vi "Confirm Hardware Found.vi"(8 "error in":errorcluster, 11 "HW Config":T1) -> (0 "error out":errorcluster, 3 "Configure Hardware?":bool)   [LabVIEW 2020, in "SEECD System Explorer.lvlib"]
uses:
  SEECD System Explorer.lvlib
  Type Defs/Host - HW Config.ctl
  Type Defs/Host - Local Chassis.ctl
  Type Defs/Host - Module.ctl
  Type Defs/IOV Container Contents.ctl
  Type Defs/Host - Master.ctl
  Type Defs/Host - Slave.ctl
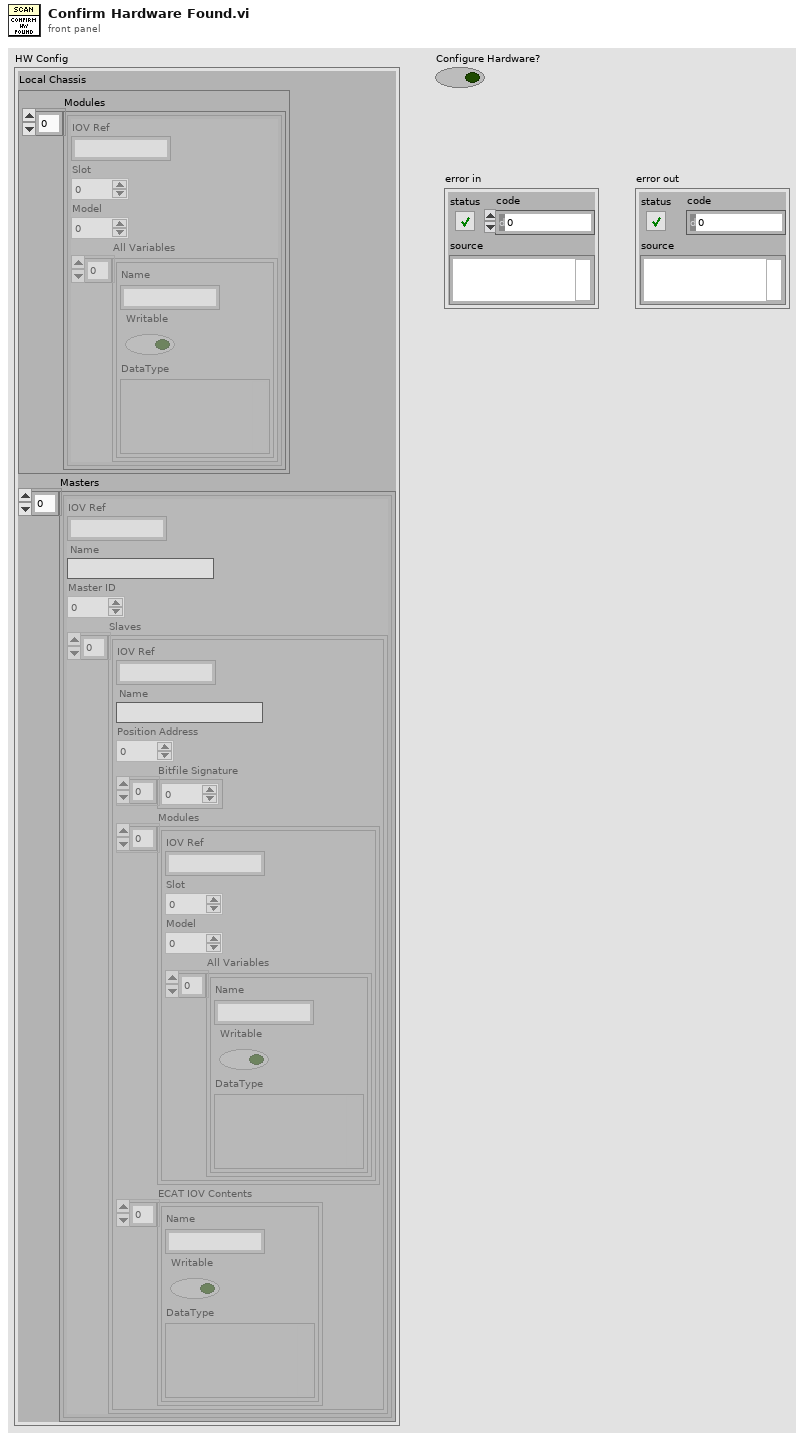
[diagram p1: front panel]
types:
  T1 = typedef "SEECD System Explorer.lvlib/Host - HW Config.ctl" = cluster{"Local Chassis":T2, "Masters":T5[]}
  T2 = typedef "SEECD System Explorer.lvlib/Host - Local Chassis.ctl" = cluster{"Modules":T3[]}
  T3 = typedef "SEECD System Explorer.lvlib/Host - Module.ctl" = cluster{"IOV Ref":string, "Slot":u32, "Model":u32, "All Variables":T4[]}
  T4 = typedef "SEECD System Explorer.lvlib/IOV Container Contents.ctl" = cluster{"Name":string, "Writable":bool, "DataType":variant}
  T5 = typedef "SEECD System Explorer.lvlib/Host - Master.ctl" = cluster{"IOV Ref":string, "Name":string, "Master ID":u32, "Slaves":T6[]}
  T6 = typedef "SEECD System Explorer.lvlib/Host - Slave.ctl" = cluster{"IOV Ref":string, "Name":string, "Position Address":u16, "Bitfile Signature":u8[], "Modules":T3[], "ECAT IOV Contents":T4[]}
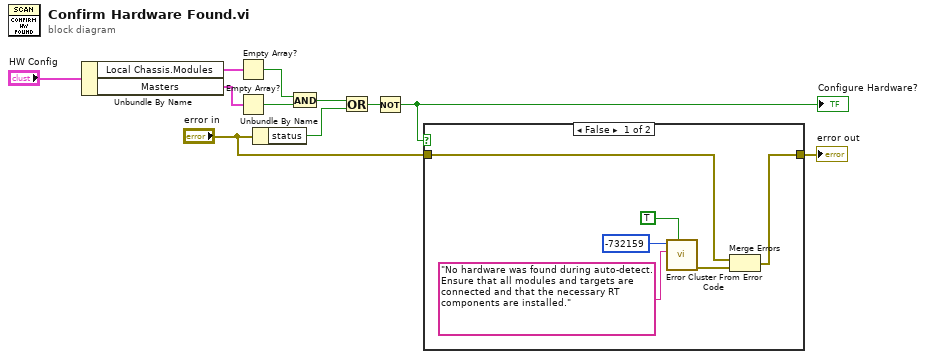
[diagram p0: block diagram]
diagram:
  n1 = Unbundle By Name("HW Config") -> ("Local Chassis.Modules"=w11:T3[], "Masters"=w9:T5[])
  n2 = Empty Array?(array=w11) -> (empty?=w8:bool)
  n3 = Empty Array?(array=w9) -> (empty?=w7:bool)
  n4 = Unbundle By Name("error in") -> ("status"=w1:bool)
  n5 = And(x=w8, y=w7) -> (x .and. y?=w6:bool)
  n6 = Or(x=w6, y=w1) -> (x .or. y?=w3:bool)
  n7 = Not(x=w3) -> (.not. x?=w2:bool)
  "Configure Hardware?" <- w2
  n8 = case shown="False" w2 {
    tunnel: "error in" -> [w14 w18]
    tunnel: [w12 w18] -> w4
    frame False {
      n9 = call <vilib>:"Error Cluster From Error Code.vi"("show call chain? (False)"=TRUE, "error message (\"\")"="No hardware was found during auto-detect. Ensure that all modules and targets are connected and that the necessary RT components are installed." ("source"), "error code (0)"=-732159 ("code")) -> ("error out"=w13:errorcluster)  [unwired: 6 in]
      n10 = Merge Errors(w14, w13) -> (w12:errorcluster)
    }
    frame True {
    }
  }
  "error out" <- w4
